vi "Show component statuses.vi"(8 "error in (no error)":errorcluster, 11 "ServiceManager in":refnum<class "ServiceManager.lvclass">) -> (0 "error out":errorcluster, 3 "ServiceManager out":refnum<class "ServiceManager.lvclass">)   [LabVIEW 2012, in "ServiceManager.lvclass"]
uses:
  ServiceManager.lvclass
  ServiceManager.lvclass/ServiceManager.ctl
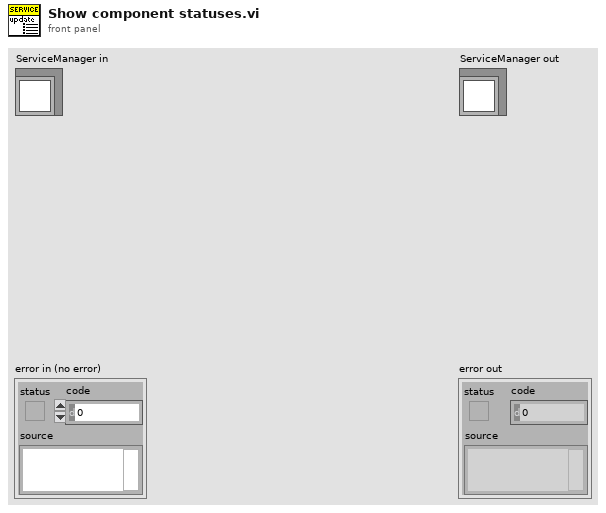
[diagram p1: front panel]
types:
  T1 = typedef "ServiceManager.lvclass/loaded_components_cluster.ctl" = cluster{"component specification":T2, "booted?":bool, "status":T3, "last seen?":timestamp}
  T2 = typedef "Murmex.lvlib/Murmex.lvclass/component_specification_cluster.ctl" = cluster{"name":string, "language":string, "host name":string, "id":string}
  T3 = typedef "Murmex.lvlib/Murmex.lvclass/status_enum.ctl" = enum16{"ready", "warning", "error", "shutting down", "initialising"}
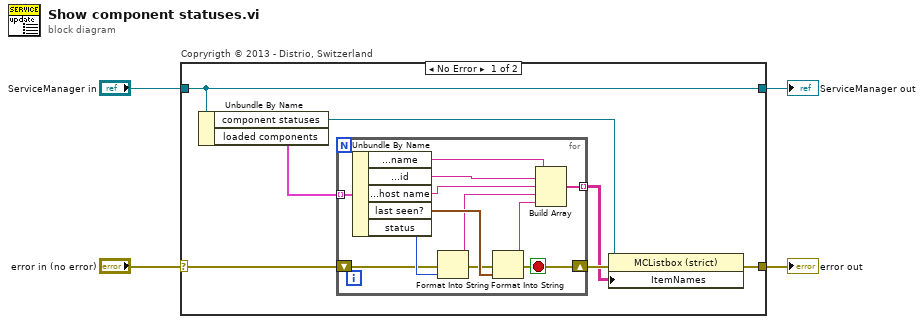
[diagram p0: block diagram]
diagram:
  n1 = case "Copryrigth © 2013 - Distrio, Switzerland" shown="No Error" "error in (no error)" {
    selector: "error in (no error)" -> [w10 w25]
    tunnel: [w6 w25] -> w3
    tunnel: [w11 w24] -> w1
    tunnel: "ServiceManager in" -> [w11 w24]
    frame No Error {
      n2 = Unbundle By Name(w11) -> ("component statuses"=w8:refnum<vi>, "loaded components"=w9:T1[])
      n3 = for {
        tunnel: w9 -> [w23] mode=indexing
        tunnel: [w18] -> w5 mode=indexing
        shift-right: [w13] -> w7
        shift-left: w10 -> [w17]
        stop <- w13 stop-if-true
        n4 = Unbundle By Name(w23) -> ("component specification.name"=w20:string, "component specification.id"=w21:string, "component specification.host name"=w12:string, "last seen?"=w22:timestamp, "status"=w19:T3)
        n5 = Format Into String(error in=w17, w19) -> (resulting string=w14:string, error out=w16:errorcluster)  [unwired: 2 in]
        n6 = Format Into String(error in=w16, w22) -> (resulting string=w15:string, error out=w13:errorcluster)  [unwired: 2 in]
        n7 = Build Array(w20, w21, w12, w14, w15) -> (w18:string[])
      }
      n8 = property class="MCListbox (strict)"(reference=w8, error in=w7, "ItemNames"=w5) -> (error out=w6:errorcluster)  [unwired: 1 out]
    }
    frame Error {
    }
  }
  "error out" <- w3
  "ServiceManager out" <- w1
